vi "LEP_RV_ConfigGlobals.vi"() -> ()   [LabVIEW 2011]
panel:
  in  "Secure connection":bool
  in  "globals set":bool
  in  "remember password":bool
  in  "password":string
  in  "username":string
  in  "server name":string
  in  "use network compile":bool
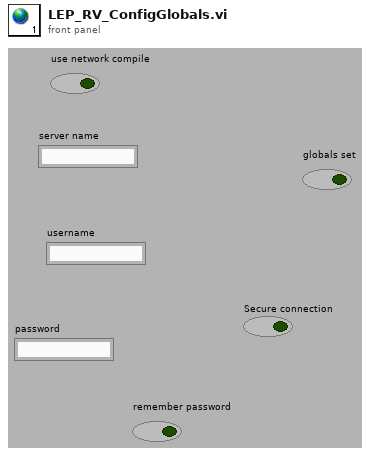
[diagram p1: front panel]
diagram:
